vi "PDash Branding.vi"(11 "This VI":refnum<vi>) -> ()   [LabVIEW 2020, in "Panther Dashboard.lvlib"]
uses:
  Panther Dashboard.lvlib
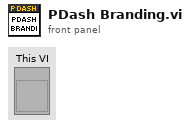
[diagram p1: front panel]
types:
  T1 = typedef "Panther Dashboard.lvlib/Pdash Style--cluster.ctl" = cluster{"Gris Obscuro Azul":u32, "Gris Medio Azul":u32, "Gris Claro Azul":u32, "Amarillo":u32, "Text color":u32, "Transparent":u32, "Fuente":string, "Text.Font:Size":u32}
  T2 = enum32{"not a typedef", "typedef", "strict typedef", "class private data"}
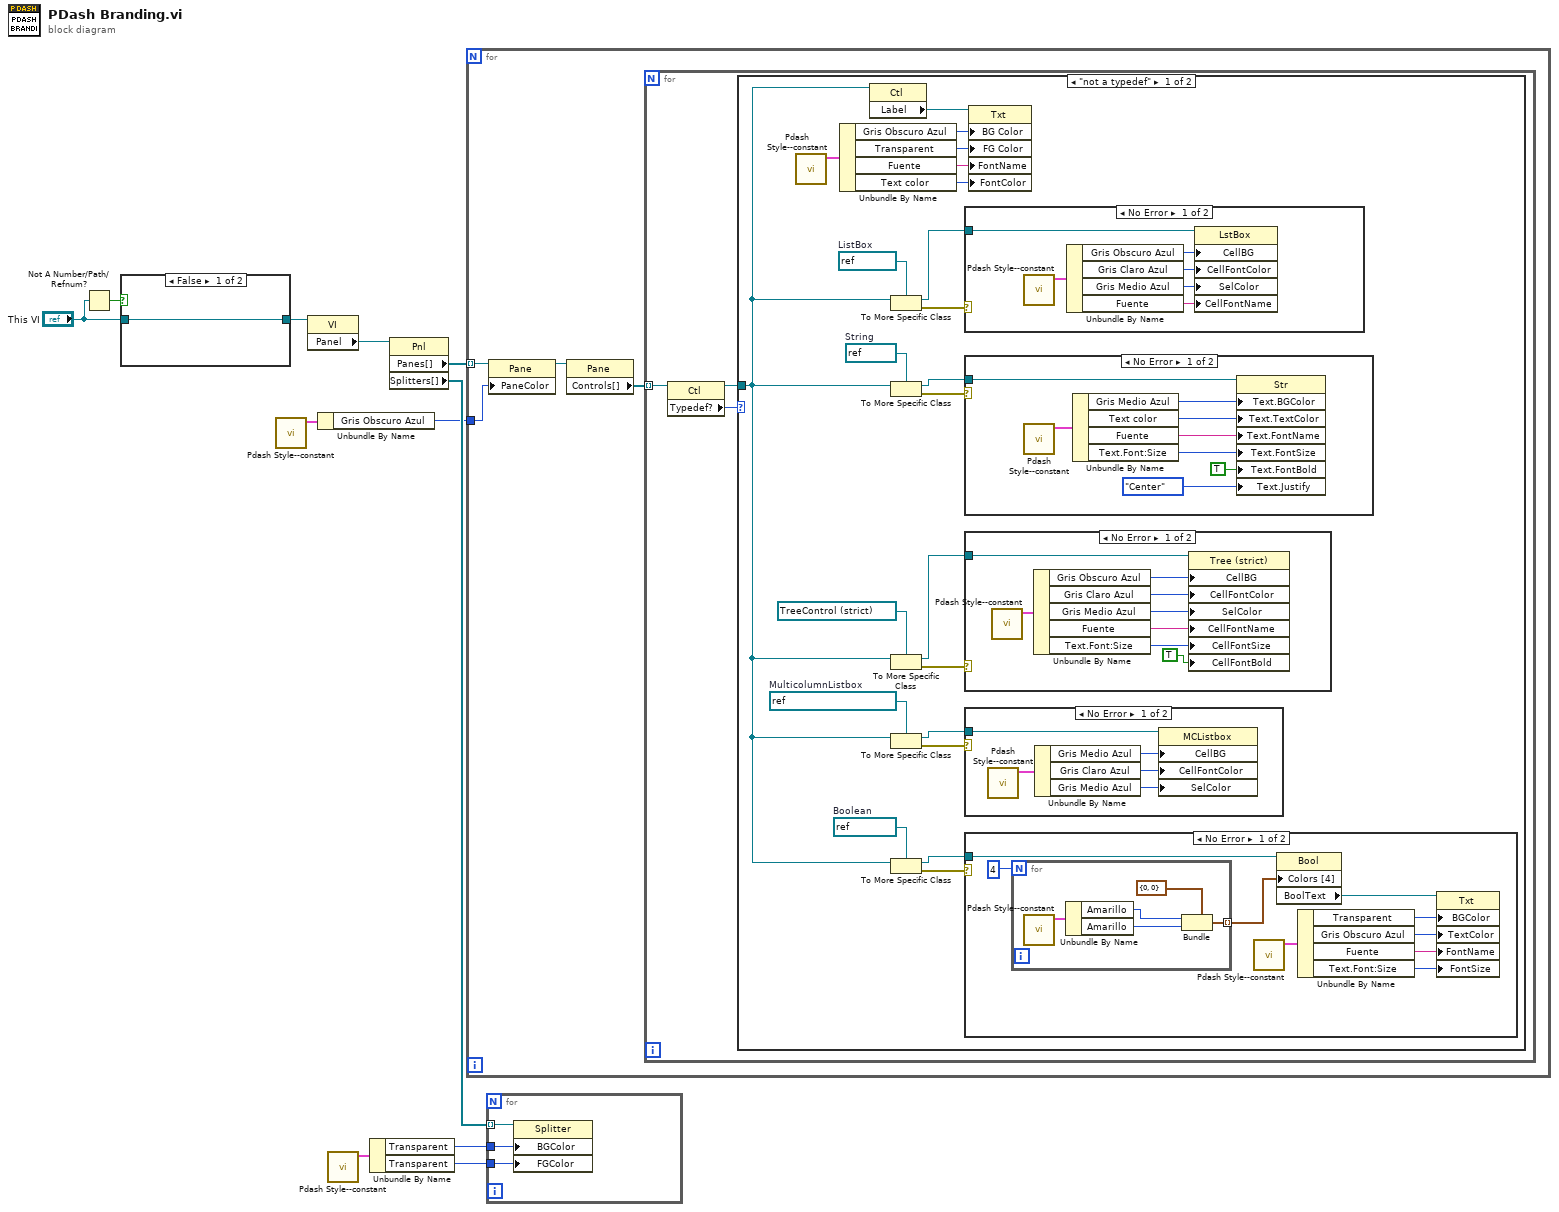
[diagram p0: block diagram]
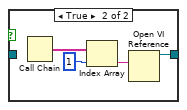
[diagram p8: hidden frame]
diagram:
  n1 = Not A Number/Path/Refnum?(number/path/refnum="This VI") -> (NaN/Path/Refnum?=w11:bool)
  n2 = case shown="False" w11 {
    tunnel: [w12 w13] -> w9
    tunnel: "This VI" -> [w12 _]
    frame False {
    }
    frame True {
      n3 = Call Chain() -> (call chain=w16:string[])
      n4 = Index Array(array=w16, index=1) -> (element=w14:string)
      n5 = Open VI Reference(vi path=w14) -> (vi reference=w13:refnum<vi>)  [unwired: 5 in, 1 out]
    }
  }
  n6 = call "Pdash Style--constant.vi"() -> ("Style"=w2:T1)  [unwired: 11 in]
  n7 = property class="VI"(reference=w9) -> ("Panel"=w8:refnum<vi>)  [unwired: 1 in, 2 out]
  n8 = Unbundle By Name(w2) -> ("Gris Obscuro Azul"=w1:u32)
  n9 = call "Pdash Style--constant.vi"() -> ("Style"=w5:T1)  [unwired: 11 in]
  n10 = Unbundle By Name(w5) -> ("Transparent"=w4:u32, "Transparent"=w3:u32)
  n11 = property class="Pnl"(reference=w8) -> ("Panes[]"=w7:refnum<vi>[], "Splitters[]"=w6:refnum<vi>[])  [unwired: 1 in, 2 out]
  n12 = for {
    tunnel: w7 -> [w20] mode=indexing
    tunnel: w1 -> [w17]
    n13 = property class="Pane"(reference=w20, "PaneColor"=w17) -> (reference out=w19:refnum<vi>)  [unwired: 1 in, 1 out]
    n14 = property class="Pane"(reference=w19) -> ("Controls[]"=w18:refnum<vi>[])  [unwired: 1 in, 2 out]
    n15 = for {
      tunnel: w18 -> [w23] mode=indexing
      n16 = property class="Ctl"(reference=w23) -> (reference out=w22:refnum<vi>, "Typedef?"=w21:T2)  [unwired: 1 in, 1 out]
      n17 = case shown="\"not a typedef\"" w21 {
        tunnel: w22 -> [w24 _]
        frame "not a typedef" {
          w33 = refnum<vi> refnum  # String
          w34 = refnum<vi> refnum  # MulticolumnListbox
          w37 = refnum<vi> refnum  # ListBox
          w39 = refnum<vi> refnum  # Boolean
          n18 = call "Pdash Style--constant.vi"() -> ("Style"=w30:T1)  [unwired: 11 in]
          n19 = Unbundle By Name(w30) -> ("Gris Obscuro Azul"=w29:u32, "Transparent"=w26:u32, "Fuente"=w28:string, "Text color"=w27:u32)
          n20 = property class="Ctl"(reference=w24) -> ("Label"=w31:refnum<vi>)  [unwired: 1 in, 2 out]
          n21 = To More Specific Class(target class=w37, reference=w24) -> (specific class reference=w36:refnum<vi>, error out=w43:errorcluster)  [unwired: 1 in]
          n22 = To More Specific Class(target class=w33, reference=w24) -> (specific class reference=w32:refnum<vi>, error out=w41:errorcluster)  [unwired: 1 in]
          n23 = To More Specific Class(target class=refnum<vi> refnum ("Tree Control"), reference=w24) -> (specific class reference=w38:refnum<vi>, error out=w44:errorcluster)  [unwired: 1 in]
          n24 = To More Specific Class(target class=w34, reference=w24) -> (specific class reference=w35:refnum<vi>, error out=w42:errorcluster)  [unwired: 1 in]
          n25 = To More Specific Class(target class=w39, reference=w24) -> (specific class reference=w40:refnum<vi>, error out=w45:errorcluster)  [unwired: 1 in]
          n26 = case shown="No Error" w43 {
            tunnel: w36 -> [w86 _]
            frame No Error {
              n27 = call "Pdash Style--constant.vi"() -> ("Style"=w85:T1)  [unwired: 11 in]
              n28 = Unbundle By Name(w85) -> ("Gris Obscuro Azul"=w84:u32, "Gris Claro Azul"=w83:u32, "Gris Medio Azul"=w82:u32, "Fuente"=w81:string)
              n29 = property class="LstBox"(reference=w86, "CellBG"=w84, "CellFontColor"=w83, "SelColor"=w82, "CellFontName"=w81) -> ()  [unwired: 1 in, 2 out]
            }
            frame Error {
            }
          }
          n30 = case shown="No Error" w41 {
            tunnel: w32 -> [w53 _]
            frame No Error {
              n31 = call "Pdash Style--constant.vi"() -> ("Style"=w52:T1)  [unwired: 11 in]
              n32 = Unbundle By Name(w52) -> ("Gris Medio Azul"=w51:u32, "Text color"=w50:u32, "Fuente"=w49:string, "Text.Font:Size"=w48:u32)
              n33 = property class="Str"(reference=w53, "Text.BGColor"=w51, "Text.TextColor"=w50, "Text.FontName"=w49, "Text.FontSize"=w48, "Text.FontBold"=TRUE ("Text.Font:Bold"), "Text.Justify"=enum16{"Left", "Center", "Right"}."Center" ("Text.Justification")) -> ()  [unwired: 1 in, 2 out]
            }
            frame Error {
            }
          }
          n34 = case shown="No Error" w44 {
            tunnel: w38 -> [w61 _]
            frame No Error {
              n35 = call "Pdash Style--constant.vi"() -> ("Style"=w66:T1)  [unwired: 11 in]
              n36 = Unbundle By Name(w66) -> ("Gris Obscuro Azul"=w65:u32, "Gris Claro Azul"=w64:u32, "Gris Medio Azul"=w63:u32, "Fuente"=w62:string, "Text.Font:Size"=w60:u32)
              n37 = property class="Tree (strict)"(reference=w61, "CellBG"=w65, "CellFontColor"=w64, "SelColor"=w63, "CellFontName"=w62, "CellFontSize"=w60, "CellFontBold"=TRUE ("Active Cell:Cell Font:Bold")) -> ()  [unwired: 1 in, 2 out]
            }
            frame Error {
            }
          }
          n38 = case shown="No Error" w42 {
            tunnel: w35 -> [w58 _]
            frame No Error {
              n39 = call "Pdash Style--constant.vi"() -> ("Style"=w57:T1)  [unwired: 11 in]
              n40 = Unbundle By Name(w57) -> ("Gris Medio Azul"=w56:u32, "Gris Claro Azul"=w55:u32, "Gris Medio Azul"=w54:u32)
              n41 = property class="MCListbox"(reference=w58, "CellBG"=w56, "CellFontColor"=w55, "SelColor"=w54) -> ()  [unwired: 1 in, 2 out]
            }
            frame Error {
            }
          }
          n42 = case shown="No Error" w45 {
            tunnel: w40 -> [w69 _]
            frame No Error {
              n43 = for {
                N: 4 -> [_]
                tunnel: [w79] -> w74 mode=indexing
                n44 = call "Pdash Style--constant.vi"() -> ("Style"=w78:T1)  [unwired: 11 in]
                n45 = Unbundle By Name(w78) -> ("Amarillo"=w76:u32, "Amarillo"=w77:u32)
                n46 = Bundle(cluster=cluster{u32, u32} {0, 0} ("Colors [4]"), w76, w77) -> (w79:cluster{u32, u32})
              }
              n47 = call "Pdash Style--constant.vi"() -> ("Style"=w72:T1)  [unwired: 11 in]
              n48 = property class="Bool"(reference=w69, "Colors [4]"=w74) -> ("BoolText"=w75:refnum<vi>)  [unwired: 1 in, 2 out]
              n49 = Unbundle By Name(w72) -> ("Transparent"=w71:u32, "Gris Obscuro Azul"=w70:u32, "Fuente"=w68:string, "Text.Font:Size"=w67:u32)
              n50 = property class="Txt"(reference=w75, "BGColor"=w71, "TextColor"=w70, "FontName"=w68, "FontSize"=w67) -> ()  [unwired: 1 in, 2 out]
            }
            frame Error {
            }
          }
          n51 = property class="Txt"(reference=w31, "BG Color"=w29, "FG Color"=w26, "FontName"=w28, "FontColor"=w27) -> ()  [unwired: 1 in, 2 out]
        }
        frame "typedef", Default {
        }
      }
    }
  }
  n52 = for {
    tunnel: w6 -> [w89] mode=indexing
    tunnel: w4 -> [w88]
    tunnel: w3 -> [w87]
    n53 = property class="Splitter"(reference=w89, "BGColor"=w88, "FGColor"=w87) -> ()  [unwired: 1 in, 2 out]
  }
